vi "Process - Remove.vi"(0 "Module Data In":T1, 11 "error in (no error)":errorcluster) -> (4 "Module Data Out":T1, 15 "error out":errorcluster)   [LabVIEW 2020, in "Template.lvlib"]
doc: "Removes from the array the current process the Module has gone through"
uses:
  Template.lvlib
  Controls/Module - Data.ctl
  Modules.ctl
  Controls/Module - States.ctl
  Controls/Timing - Data.ctl
  Controls/Process - Element.ctl
  Controls/Process.ctl
  Controls/Process - Status.ctl
  Error Handler - Logger Module/Error Handler - Logger.lvlib
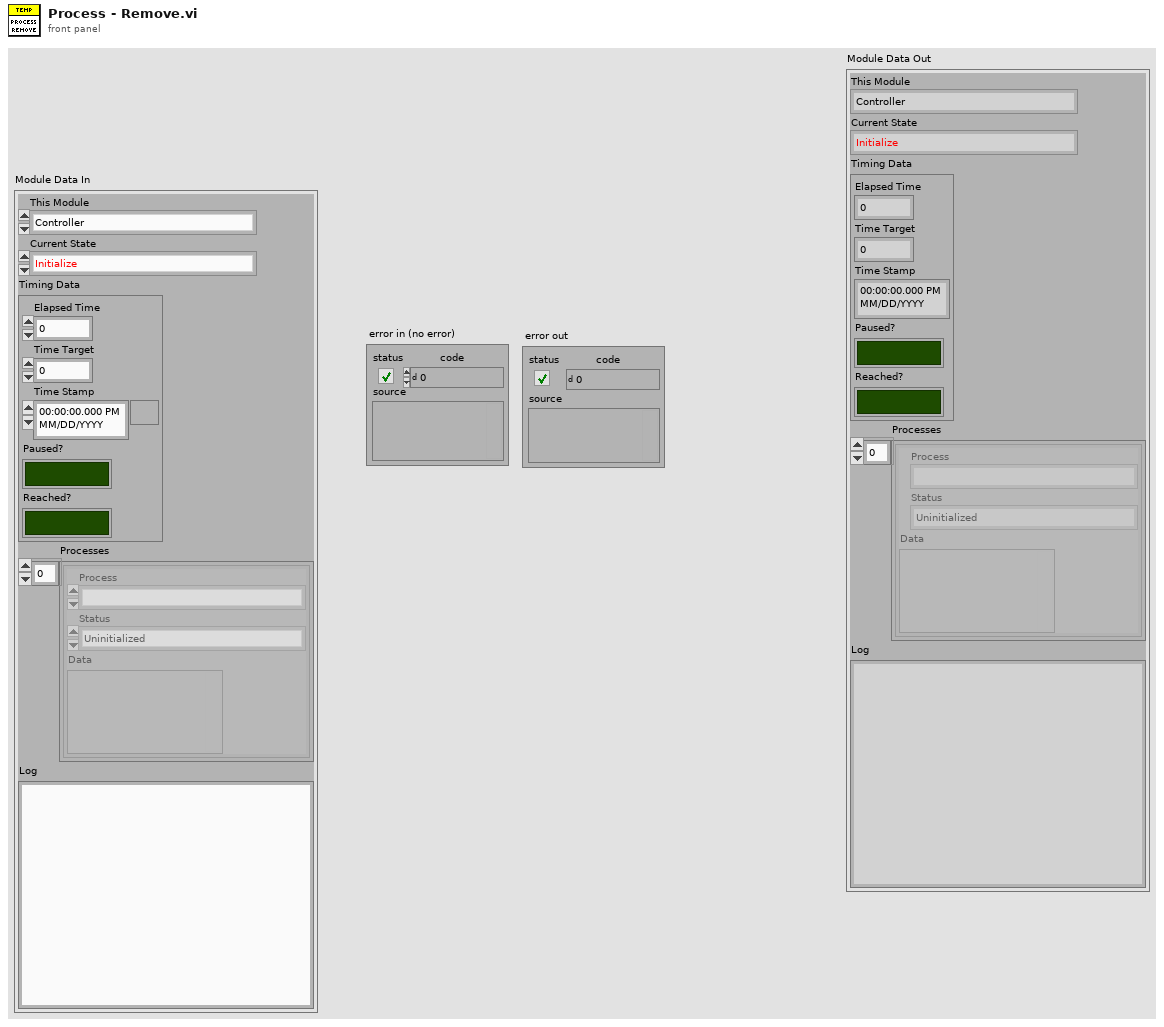
[diagram p1: front panel]
types:
  T1 = typedef "Template.lvlib/Module - Data.ctl" = cluster{"This Module":T2, "Current State":T3, "Timing Data":T4, "Processes":T5[], "Log":string}
  T2 = typedef "Error Handler - Logger.lvlib/Modules.ctl" = enum16{"Controller", "Error Handler - Logger"}
  T3 = typedef "Template.lvlib/Module - States.ctl" = enum16{"Initialize", "Event ", "Send data", "FP Element: Update", "FP Element: Disable/Enable", "Timer: Setup", "Terminate", "---------------Template---------------"}
  T4 = typedef "Template.lvlib/Timing - Data.ctl" = cluster{"Elapsed Time":dbl, "Time Target":dbl, "Time Stamp":timestamp, "Paused?":bool, "Reached?":bool}
  T5 = typedef "Template.lvlib/Process - Element.ctl" = cluster{"Process":T6, "Status":T7, "Data":variant}
  T6 = typedef "Template.lvlib/Process.ctl" = enum16{""}
  T7 = typedef "Template.lvlib/Process - Status.ctl" = enum16{"Uninitialized", "Busy"}
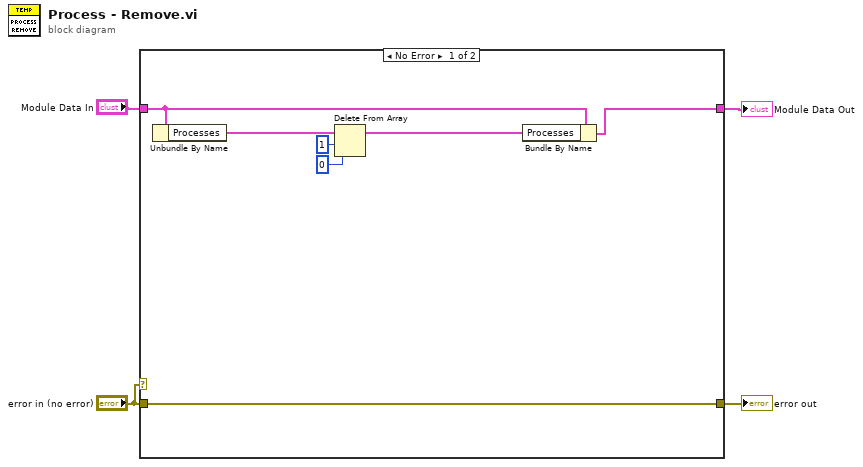
[diagram p0: block diagram]
diagram:
  n1 = case shown="No Error" "error in (no error)" {
    tunnel: [w9 w13] -> w4
    tunnel: "Module Data In" -> [w10 w13]
    tunnel: [w11 w12] -> w2
    tunnel: "error in (no error)" -> [w11 w12]
    frame No Error {
      n2 = Unbundle By Name(w10) -> ("Processes"=w8:T5[])
      n3 = Delete From Array(array=w8, length=1, index=0) -> (array with subset deleted=w7:T5[])  [unwired: 1 out]
      n4 = Bundle By Name(cluster=w10, "Processes"=w7) -> (w9:T1)
    }
    frame Error {
    }
  }
  "error out" <- w2
  "Module Data Out" <- w4
